vi "Tag Viewer.vi"() -> ()   [LabVIEW 2015]
uses:
  <vilib>/TagLibrary/Read Double Values.vi
  <vilib>/TagLibrary/Tag Library.lvlib
  <resource>/objmgr/niTag.rc
panel:
  out "Number of tags":i32
  out "Tags":string[][](table)
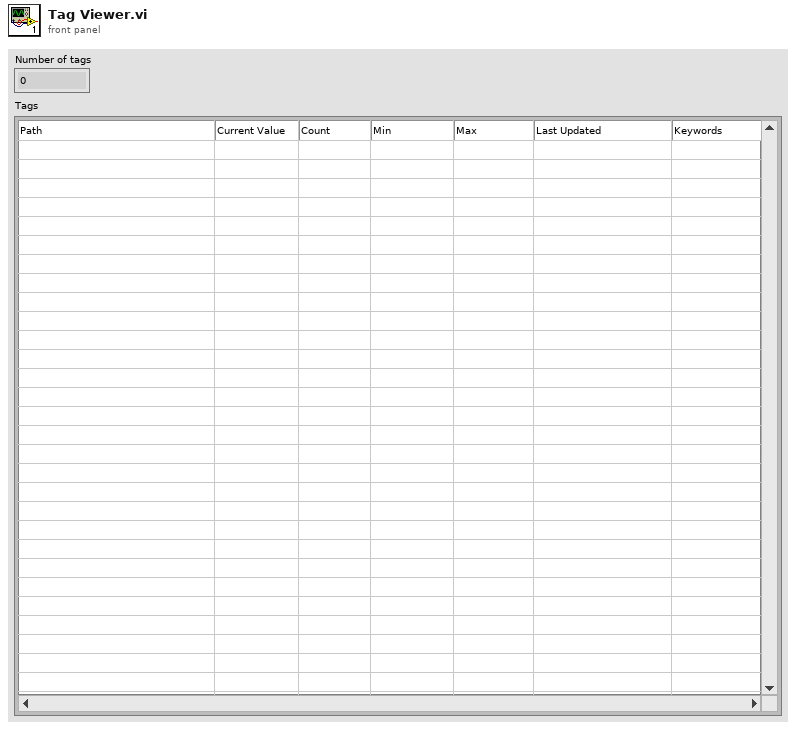
[diagram p1: front panel]
types:
  T1 = typedef "Tag Library.lvlib/Aggregates Double.ctl" = cluster{"count":i32, "max":dbl, "min":dbl, "sum":dbl, "mean":dbl}
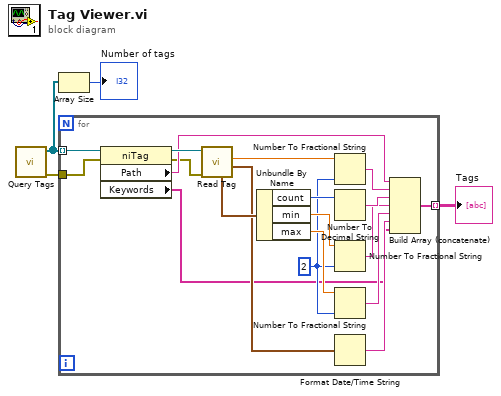
[diagram p0: block diagram]
diagram:
  n1 = call <vilib>:"Query Tags.vi"() -> ("error out"=w1:errorcluster, "query results (references)"=w3:refnum<k21>[])  [unwired: 10 in]
  n2 = Array Size(array=w3) -> (size(s)=→"Number of tags":i32)
  n3 = for {
    tunnel: w3 -> [w22] mode=indexing
    tunnel: [w10] -> w2 mode=indexing
    tunnel: w1 -> [w6]
    w9 = i16 2 ("precision (6)")
    n4 = property class="niTag"(reference=w22, error in=w6) -> (reference out=w21:refnum<k21>, error out=w5:errorcluster, "Path"=w15:string, "Keywords"=w7:string[])
    n5 = call-poly <vilib>:"Read Tag.vi"("error in (no error)"=w5, "tag reference (in)"=w21) -> ("timestamp"=w19:timestamp, "double"=w20:dbl, "Aggregates (Double)"=w23:T1)  [unwired: 5 in, 2 out]
    n6 = Unbundle By Name(w23) -> ("count"=w18:i32, "min"=w17:dbl, "max"=w16:dbl)
    n7 = Number To Fractional String(number=w20, precision (6)=w9) -> (F-format string=w14:string)  [unwired: 2 in]
    n8 = Number To Decimal String(number=w18) -> (decimal integer string=w13:string)  [unwired: 1 in]
    n9 = Number To Fractional String(number=w17, precision (6)=w9) -> (F-format string=w12:string)  [unwired: 2 in]
    n10 = Number To Fractional String(number=w16, precision (6)=w9) -> (F-format string=w11:string)  [unwired: 2 in]
    n11 = Format Date/Time String(seconds (now)=w19) -> (date/time string=w8:string)  [unwired: 2 in]
    n12 = Build Array (concatenate)(w15, w14, w13, w12, w11, w8, w7) -> (w10:string[])
  }
  "Tags" <- w2
